vi "Range.vi"() -> (0 "Center":i32, 3 "NumBins":i32)   [LabVIEW 2019]
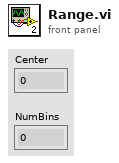
[diagram p1: front panel]
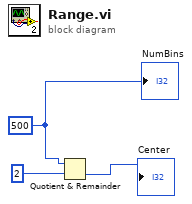
[diagram p0: block diagram]
diagram:
  w3 = 500
  n1 = Quotient & Remainder(x=w3, y=2) -> (floor(x/y)=→"Center":i32)  [unwired: 1 out]
  "NumBins" <- w3
